vi "UR3_IK.vi"(0 "Transformation Matrix":T1, 1 "Max Iterations":i32=100, 2 "guess (deg)":sgl[](array[numeric])=[0.0, 0.0, 0.0, 0.0, 0.0, 0.0], 3 "Threshold":dbl=1e-05) -> (5 "3D Picture":refnum<vi>(3d-picture), 6 "q (deg)":dbl[](array[numeric]), 7 "iterations":i32)   [LabVIEW 2024]
uses:
  <vilib>/Analysis/Matrix/Datatypes/RealMatrix.ctl
  <vilib>/Analysis/Matrix/NI_Matrix.lvlib
panel:
  out "success?":bool
  out "Calculated Transformation Matrix":T1=[[1.0, 0.0, 0.0, 0.0], [0.0, 6.123233995736766e-17, 1.0, 0.0], [0.0, -1.0, 6.123233995736766e-17, 0.0], [0.0, 0.0, 0.0, 1.0]] format="%#_2g"
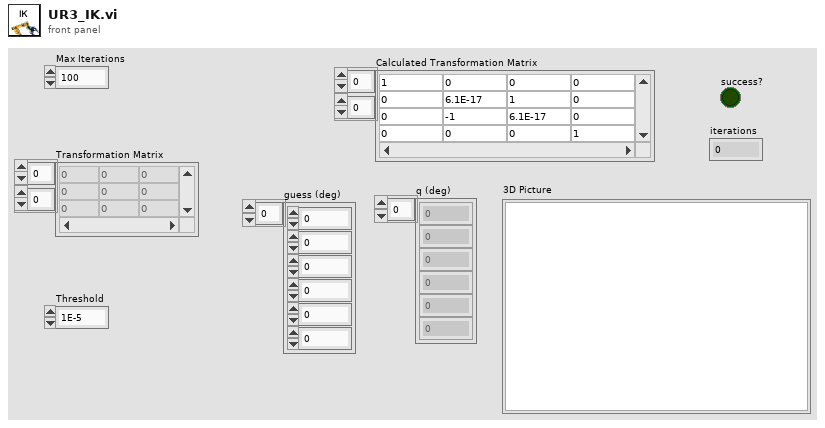
[diagram p1: front panel]
types:
  T1 = typedef "NI_Matrix.lvlib/RealMatrix.ctl" = dbl[][]
  T2 = cluster{"theta (deg)":dbl, "d":dbl, "a":dbl, "alpha (deg)":dbl}[]
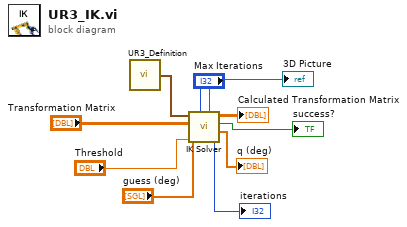
[diagram p0: block diagram]
diagram:
  n1 = call <userlib>:"UR3_Definition.vi"() -> ("UR3"=w2:T2)  [unwired: 1 in]
  n2 = call <userlib>:"IK Solver.vi"("Max Iterations"="Max Iterations", "Threshold"="Threshold", "guess (deg)"="guess (deg)", "Final Transformation Matrix"="Transformation Matrix", "Joints"=w2) -> ("iterations"=→"iterations":i32, "result (deg)"=→"q (deg)":dbl[], "success?"=→"success?":bool, "Calculated Transformation Matrix"=→"Calculated Transformation Matrix":T1, "3D Picture"=→"3D Picture":refnum<vi>)  [unwired: 2 in]
